vi "Stop.vi"(7 "Wait Until Done?":bool, 8 "error in (no error)":errorcluster, 11 "AO (Continuous) Ref In":T1) -> (0 "error out":errorcluster, 3 "AO (Continuous) Ref Out":T1)   [LabVIEW 2021, in "AO Continuous.lvlib"]
doc: "Stops signal generation on the FPGA target."
uses:
  <vilib>/myRIO/Instrument Drivers/Onboard IO/AO Continuous/AO Continuous.lvlib
  <vilib>/myRIO/Instrument Drivers/Onboard IO/AO Continuous/typedefs/AO Continuous Reference.ctl
  <vilib>/myRIO/Common/Instrument Driver Framework/Utilities/typedefs/myRIO Generic Hardware Reference.ctl
  <vilib>/myRIO/Common/Instrument Driver Framework/Utilities/typedefs/Hardware Version Enum.ctl
  <vilib>/myRIO/Common/Instrument Driver Framework/Utilities/typedefs/myRIO v1.0 Reference.ctl
  <vilib>/myRIO/Common/Instrument Driver Framework/Utilities/typedefs/Generic FPGA Reference.ctl
  <vilib>/myRIO/Common/Instrument Driver Framework/ELVIS III v1.0/AO Continuous/typedefs/AO Continuous Channels List.ctl
  <vilib>/myRIO/Common/Instrument Driver Framework/ELVIS III v1.0/AO Continuous/typedefs/ELVIS III v1.0 AO Continuous Channels Enum.ctl
  <vilib>/myRIO/Common/Instrument Driver Framework/ELVIS III v1.0/AO Continuous/typedefs/AO Continuous Channel Info.ctl
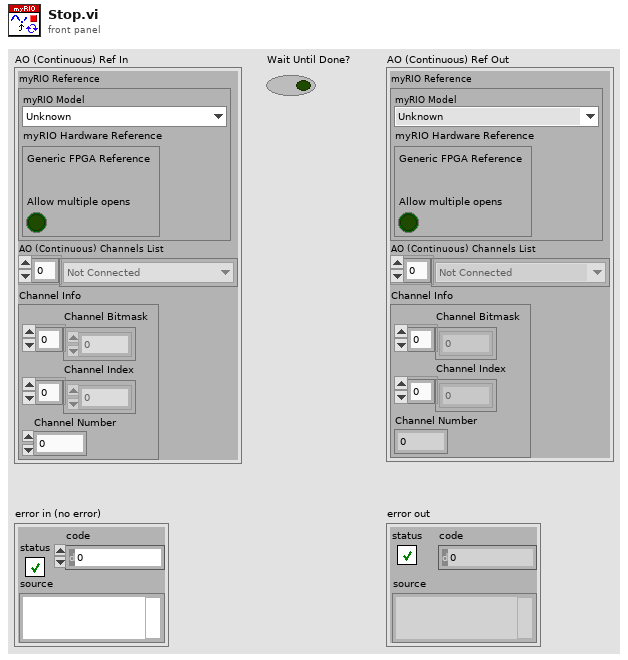
[diagram p1: front panel]
types:
  T1 = typedef "AO Continuous.lvlib/AO Continuous Reference.ctl" = cluster{"myRIO Reference":T2, "AO (Continuous) Channels List":T6, "Channel Info":T8}
  T2 = typedef "myRIO Generic Hardware Reference.ctl" = cluster{"myRIO Model":T3, "myRIO Hardware Reference":T4}
  T3 = typedef "Hardware Version Enum.ctl" = enum16{"Unknown", "myRIO-1900", "myRIO-1950", "roboRIO", "NI ELVIS RIO CM", "ELVIS III"}
  T4 = typedef "myRIO v1.0 Reference.ctl" = cluster{"Generic FPGA Reference":T5, "Allow multiple opens":bool}
  T5 = typedef "Generic FPGA Reference.ctl" = refnum<k20>
  T6 = typedef "AO Continuous Channels List.ctl" = T7[]
  T7 = typedef "ELVIS III v1.0 AO Continuous Channels Enum.ctl" = enum16{"Not Connected", "A/AO0 (Continuous)", "A/AO1 (Continuous)", "B/AO0 (Continuous)", "B/AO1 (Continuous)"}
  T8 = typedef "AO Continuous Channel Info.ctl" = cluster{"Channel Bitmask":u8[], "Channel Index":i32[], "Channel Number":u8}
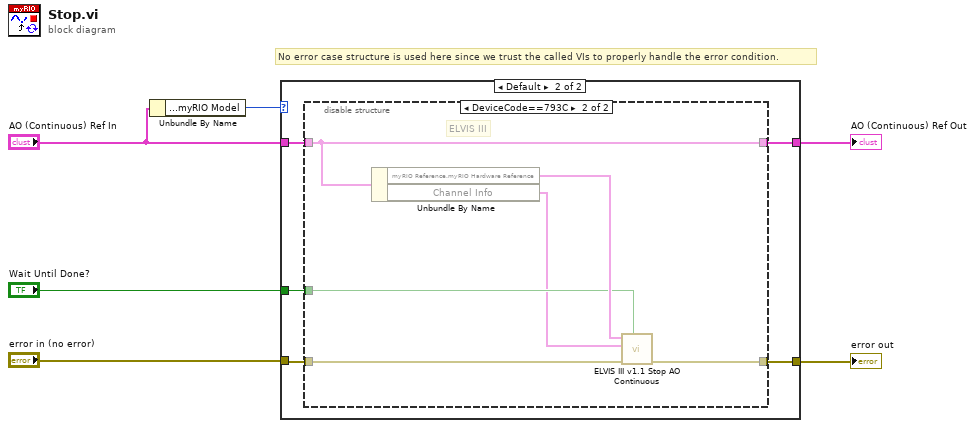
[diagram p0: block diagram]
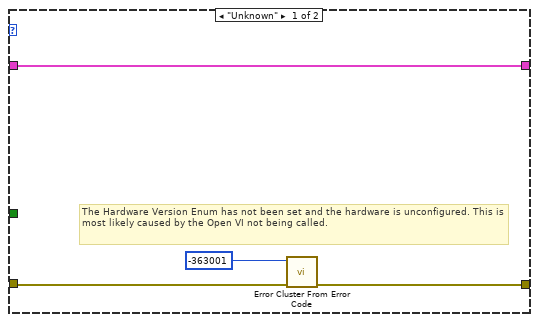
[diagram p2: hidden frame]
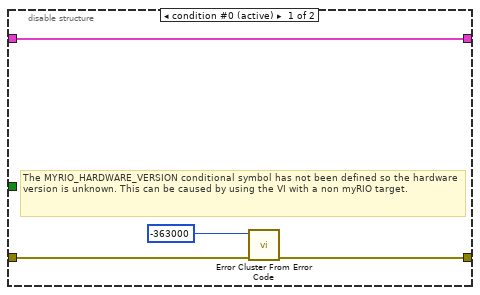
[diagram p3: hidden frame]
diagram:
  # "No error case structure is used here since we trust the called VIs to properly handle the error condition."
  n1 = Unbundle By Name("AO (Continuous) Ref In") -> ("myRIO Reference.myRIO Model"=w4:T3)
  n2 = case shown="Default" w4 {
    tunnel: [w8 w15] -> w5
    tunnel: "AO (Continuous) Ref In" -> [w7 w14]
    tunnel: "error in (no error)" -> [w9 w13]
    tunnel: [w7 w12] -> w1
    tunnel: "Wait Until Done?" -> [_ w11]
    frame "Unknown" {
      # "The Hardware Version Enum has not been set and the hardware is unconfigured. This is most likely caused by the Open VI not being called."
      n3 = call <vilib>:"Error Cluster From Error Code.vi"("error in (no error)"=w9, "error code (0)"=-363001) -> ("error out"=w8:errorcluster)  [unwired: 7 in]
    }
    frame Default {
      n4 = disable-structure shown="DeviceCode==793C" {
        disable-tunnel: w14 -> [w16 w24]
        disable-tunnel: [w19 w23] -> w15
        disable-tunnel: w13 -> [w17 w22]
        disable-tunnel: [w16 w24] -> w12
        disable-tunnel: w11 -> [_ w21]
        frame condition #0 (active) {
          # "The MYRIO_HARDWARE_VERSION conditional symbol has not been defined so the hardware version is unknown. This can be caused by using the VI with a non myRIO target."
          n5 = call <vilib>:"Error Cluster From Error Code.vi"("error in (no error)"=w17, "error code (0)"=-363000) -> ("error out"=w19:errorcluster)  [unwired: 7 in]
        }
        frame condition #1 {
          # "ELVIS III"
          n6 = Unbundle By Name(w24) -> ("myRIO Reference.myRIO Hardware Reference"=w25:T4, "Channel Info"=w20:T8)
          n7 = call <vilib>:"ELVIS III v1.1 Stop AO Continuous.vi"("Wait Until Done?"=w21, "error in (no error)"=w22, "Channel Info"=w20, "myRIO Ref In"=w25) -> ("error out"=w23:errorcluster)  [unwired: 6 in, 1 out]
        }
      }
    }
  }
  "error out" <- w5
  "AO (Continuous) Ref Out" <- w1
